vi "GetDigitalInputVals.vi"(8 "error in (no error)":errorcluster, 11 "SerialPortRef":T1) -> (0 "error out":errorcluster, 2 "All Digital Input Vals":bool[](array[boolean]), 3 "SerialPortRef 2":T1)   [LabVIEW 2015]
uses:
  <vilib>/Rock Robotics/WPI/SerialPort/WPI_SerialPortRef.ctl
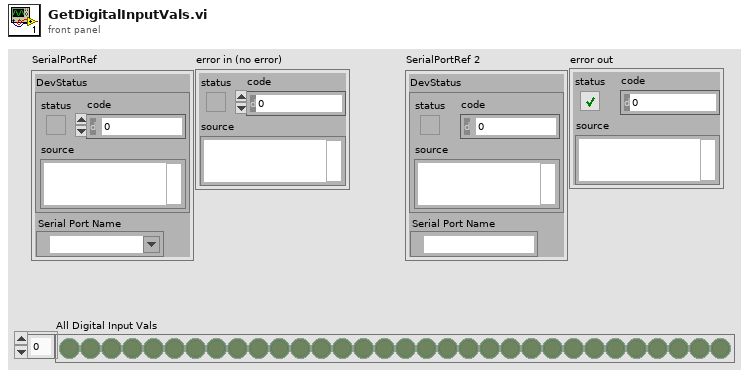
[diagram p1: front panel]
types:
  T1 = typedef "WPI_SerialPortRef.ctl" = cluster{"DevStatus":errorcluster, "Serial Port Name":refnum<visa-resource-name>}
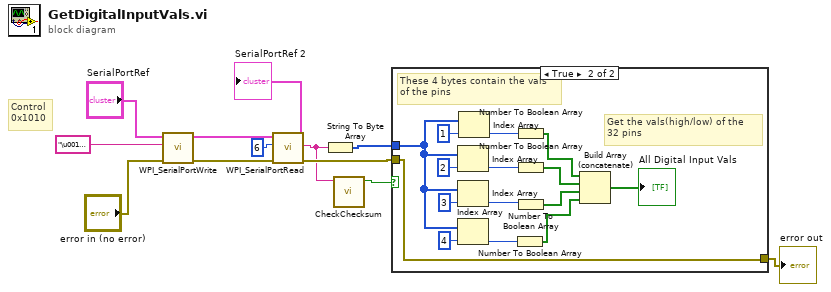
[diagram p0: block diagram]
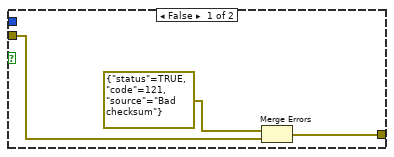
[diagram p2: hidden frame]
diagram:
  # "Control\n0x1010"
  n1 = call <vilib>:"WPI_SerialPortWrite.vi"("error in (no error)"="error in (no error)", "Buffer"="\u0010\u0010", "SerialPortRef"="SerialPortRef") -> ("error out"=w8:errorcluster, "SerialPortRef"=w9:T1)  [unwired: 6 in, 1 out]
  n2 = call <vilib>:"WPI_SerialPortRead.vi"("error in (no error)"=w8, "Num Bytes to Read"=u32 6, "SerialPortRef"=w9) -> ("error out"=w5:errorcluster, "Buffer"=w3:string, "SerialPortRef"=→"SerialPortRef 2":T1)  [unwired: 6 in]
  n3 = String To Byte Array(string=w3) -> (unsigned byte array=w1:u8[])
  n4 = call "CheckChecksum.vi"("String"=w3) -> ("x = y?"=w2:bool)  [unwired: 9 in, 1 out]
  n5 = case shown="True" w2 {
    tunnel: w1 -> [_ w17]
    tunnel: w5 -> [w14 w16]
    tunnel: [w13 w16] -> w4
    frame False {
      n6 = Merge Errors(errorcluster {"status"=TRUE, "code"=121, "source"="Bad checksum"} ("error in"), w14) -> (w13:errorcluster)
    }
    frame True {
      # "These 4 bytes contain the vals \nof the pins"
      # "Get the vals(high/low) of the \n32 pins"
      n7 = Index Array(array=w17, index=2) -> (element=w23:u8)
      n8 = Index Array(array=w17, index=3) -> (element=w24:u8)
      n9 = Index Array(array=w17, index=4) -> (element=w25:u8)
      n10 = Index Array(array=w17, index=1) -> (element=w26:u8)
      n11 = Number To Boolean Array(number=w25) -> (Boolean array=w19:bool[])
      n12 = Number To Boolean Array(number=w26) -> (Boolean array=w22:bool[])
      n13 = Number To Boolean Array(number=w23) -> (Boolean array=w21:bool[])
      n14 = Number To Boolean Array(number=w24) -> (Boolean array=w20:bool[])
      n15 = Build Array (concatenate)(w22, w21, w20, w19) -> (→"All Digital Input Vals":bool[])
    }
  }
  "error out" <- w4
